vi "DeactivateChnl HW.vi"(8 "error in (no error)":errorcluster, 10 "Chnl Name":string, 11 "BME_DG_Base in":refnum<class "BME_DG_Base.lvclass">) -> (0 "error out":errorcluster, 3 "BME_DG_Base out":refnum<class "BME_DG_Base.lvclass">)   [LabVIEW 2009, in "POLARIS BME DG.lvlib" / "BME_DG_Base.lvclass"]
uses:
  BME_DG_Base.lvclass
  BME_DG_Chnl/BME_DG_Chnl.lvclass
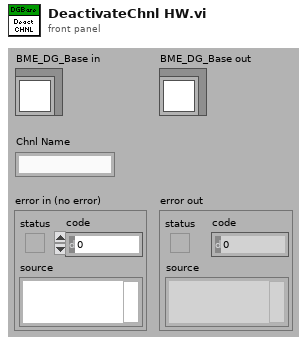
[diagram p1: front panel]
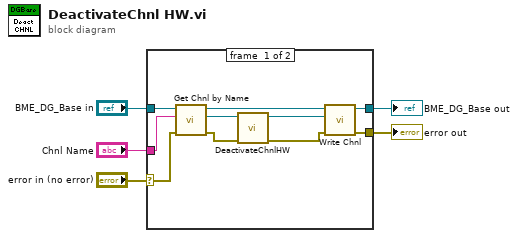
[diagram p0: block diagram]
diagram:
  n1 = case shown="No Error" "error in (no error)" {
    selector: "error in (no error)" -> [w14 w17]
    tunnel: [w7 w17] -> w4
    tunnel: [w6 w16] -> w2
    tunnel: "BME_DG_Base in" -> [w15 w16]
    tunnel: "Chnl Name" -> [w13 _]
    frame #0 {
      n2 = call-dynamic "Get Chnl by Name.vi"("error in (no error)"=w14, "Chnl Name"=w13, "BME_DG_Base in"=w15) -> ("error out"=w11:errorcluster, "BME_DG_Chnl out"=w12:refnum<class "BME_DG_Chnl.lvclass">, "BME_DG_Base out"=w10:refnum<class "BME_DG_Base.lvclass">)  [unwired: 5 in, 1 out]
      n3 = call "DeactivateChnlHW.vi"("error in (no error)"=w11, "BME_DG_Chnl in"=w12) -> ("error out"=w8:errorcluster, "BME_DG_Chnl out"=w9:refnum<class "BME_DG_Chnl.lvclass">)  [unwired: 8 in]
      n4 = call-dynamic "Write Chnl.vi"("error in (no error)"=w8, "BME_DG_Chnl"=w9, "BME_DG_Base in"=w10) -> ("error out"=w7:errorcluster, "BME_DG_Base out"=w6:refnum<class "BME_DG_Base.lvclass">)  [unwired: 7 in]
    }
    frame #1 {
    }
  }
  "error out" <- w4
  "BME_DG_Base out" <- w2
